vi "Recompose Item.vi"(8 "error in (no error)":errorcluster, 9 "Nesting Level":i32, 10 "All Data":refnum<class "Data Item.lvclass">[](array[class]), 11 "Element in":refnum<class "Element.lvclass">) -> (0 "error out":errorcluster, 1 "XML String":string, 2 "All Data out":refnum<class "Data Item.lvclass">[](array[class]), 3 "Element out":refnum<class "Element.lvclass">)   [LabVIEW 2026, in "VILab.lvlib" / "Element.lvclass"]
uses:
  Element.lvclass
  Data Item/Data Item.lvclass
  <vilib>/AdvancedString/1D String Array to Delimited String (string).vi
  VILab.lvlib
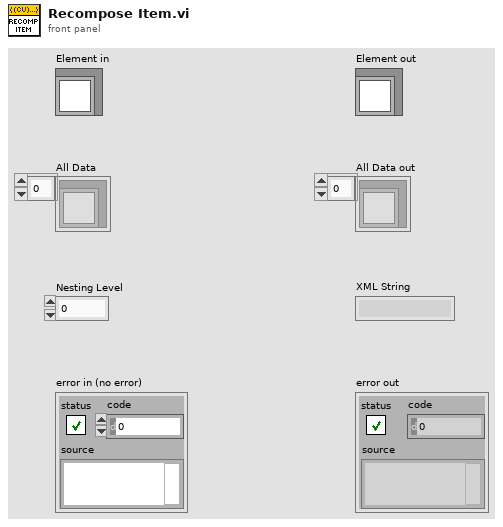
[diagram p1: front panel]
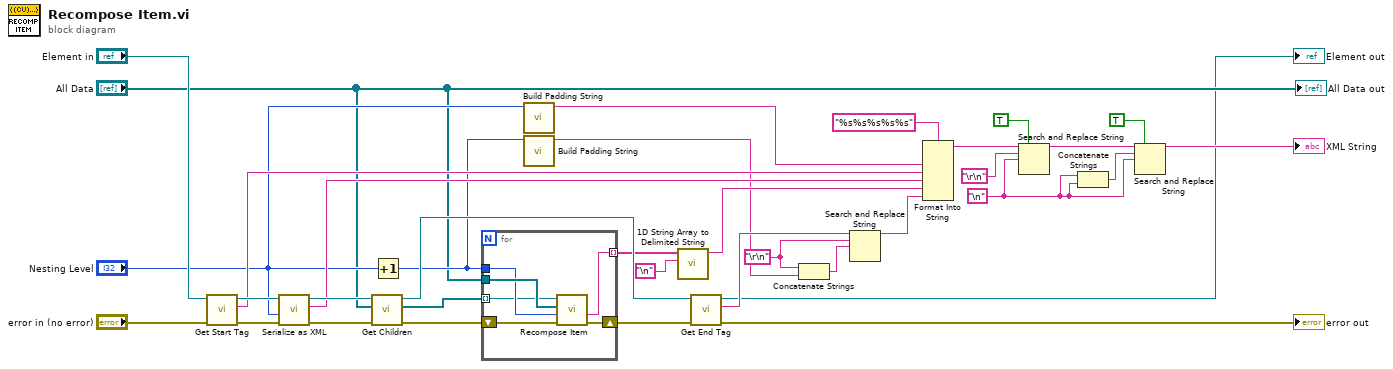
[diagram p0: block diagram]
diagram:
  w9 = "\n"
  w20 = "\r\n"
  n1 = call-dynamic "Get Start Tag.vi"("error in (no error)"="error in (no error)", "Element in"="Element in") -> ("error out"=w30:errorcluster, "Start Tag"=w26:string, "Element out"=w29:refnum<class "Element.lvclass">)  [unwired: 7 in]
  n2 = call-dynamic "Serialize as XML.vi"("error in (no error)"=w30, "Nesting Level"="Nesting Level", "Element in"=w29) -> ("error out"=w34:errorcluster, "XML Fragment"=w25:string, "Element out"=w32:refnum<class "Element.lvclass">)  [unwired: 6 in]
  n3 = call-dynamic "Get Children.vi"("error in (no error)"=w34, "All Data"="All Data", "Element in"=w32) -> ("error out"=w33:errorcluster, "Children"=w31:refnum<class "Data Item.lvclass">[], "Element out"=w28:refnum<class "Element.lvclass">)  [unwired: 5 in, 1 out]
  n4 = Increment(x="Nesting Level") -> (x+1=w16:i32)
  n5 = for {
    shift-right: [w40] -> w35
    shift-left: w33 -> [w37]
    tunnel: w31 -> [w36] mode=indexing
    tunnel: "All Data" -> [w41]
    tunnel: [w38] -> w24 mode=indexing
    tunnel: w16 -> [w39]
    n6 = call-dynamic "Recompose Item.vi"("error in (no error)"=w37, "Nesting Level"=w39, "All Data"=w41, "Data Item in"=w36) -> ("error out"=w40:errorcluster, "XML String"=w38:string)  [unwired: 4 in, 2 out]
  }
  n7 = call "Build Padding String.vi"("Nesting Level"="Nesting Level") -> ("Padding"=w17:string)  [unwired: 10 in]
  n8 = call "Build Padding String.vi"("Nesting Level"=w16) -> ("Padding"=w15:string)  [unwired: 10 in]
  n9 = call-poly <vilib>:"1D String Array to Delimited String.vi"("delimiter"="\n", "string array"=w24) -> ("delimited string"=w22:string)  [unwired: 9 in]
  n10 = call-dynamic "Get End Tag.vi"("error in (no error)"=w35, "Element in"=w28) -> ("error out"=→"error out":errorcluster, "End Tag"=w21:string, "Element out"=→"Element out":refnum<class "Element.lvclass">)  [unwired: 7 in]
  n11 = Concatenate Strings(w20, w15) -> (w19:string)
  n12 = Search and Replace String(input string=w21, search string=w20, replace string=w19) -> (result string=w18:string)  [unwired: 5 in, 3 out]
  n13 = Format Into String(format string="%s%s%s%s%s", w17, w26, w25, w22, w18) -> (resulting string=w14:string)  [unwired: 2 in, 1 out]
  n14 = Search and Replace String(replace all?=TRUE ("replace all? (F)"), input string=w14, search string="\r\n", replace string=w9) -> (result string=w10:string)  [unwired: 4 in, 3 out]
  n15 = Concatenate Strings(w9, w9) -> (w8:string)
  n16 = Search and Replace String(replace all?=TRUE ("replace all? (F)"), input string=w10, search string=w8, replace string=w9) -> (result string=→"XML String":string)  [unwired: 4 in, 3 out]
  "All Data out" <- "All Data"
